vi "Agilent N6700 Series Read External Datalog.vi"() -> ()   [LabVIEW 2016]
doc: "Configures the external datalog then reads it from the instrument's buffer."
uses:
  <instrlib>/Agilent N6700 Series/Agilent N6700 Series.lvlib
panel:
  out "External Log":string
  in  "Max Records (10)":i32=10
  in  "Enable Minimum Maximum Log (False)":bool
  in  "Enable Data Log (True)":bool=TRUE
  in  "Data Log Period (0.1 s)":dbl=0.1
  in  "Data Log Auto Range (False)":bool=TRUE
  in  "Data Log Type (1: Voltage)":i32(ring)=1 items=["Voltage"=1, "Current"=0]
  in  "Channel Name (3)":string="3"
  in  "VISA resource name":refnum<visa-resource-name>
  # "(c) 2004-2019  National Instruments.  ALL RIGHTS RESERVED."
  # "Agilent N6700 DC Power Supply"
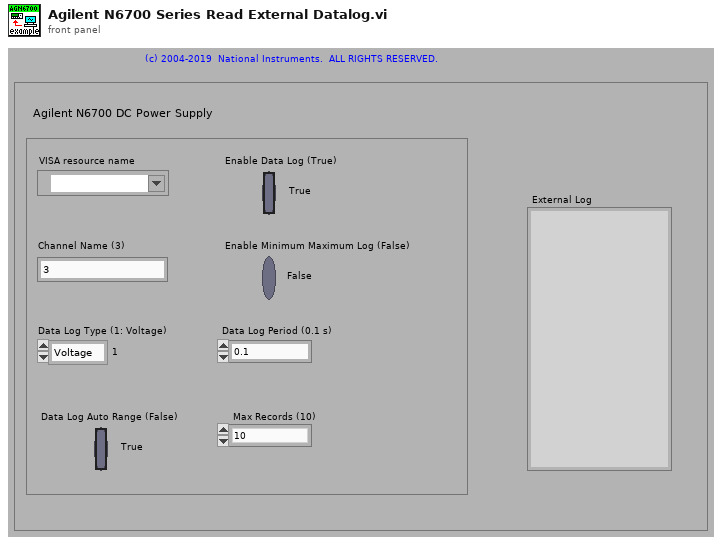
[diagram p1: front panel]
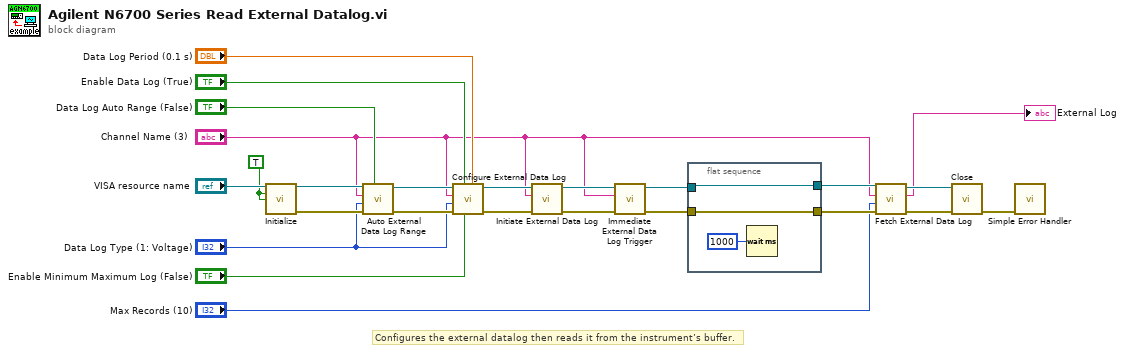
[diagram p0: block diagram]
diagram:
  w23 = TRUE ("Reset? (T: Yes)")
  # "Configures the external datalog then reads it from the instrument’s buffer."
  n1 = call <instrlib>:"Initialize.vi"("VISA resource name"="VISA resource name", "ID Query? (T: Yes)"=w23, "Reset? (T: Yes)"=w23) -> ("VISA resource name out"=w22:refnum<visa-resource-name>, "error out"=w21:errorcluster)  [unwired: 11 in]
  n2 = call <instrlib>:"Auto External Data Log Range.vi"("External Data Log Auto Range (False)"="Data Log Auto Range (False)", "error in (no error)"=w21, "External Data Log Type (1: Voltage)"="Data Log Type (1: Voltage)", "Channel Name (1)"="Channel Name (3)", "VISA resource name"=w22) -> ("error out"=w18:errorcluster, "VISA resource name out"=w19:refnum<visa-resource-name>)  [unwired: 5 in]
  n3 = call <instrlib>:"Configure External Data Log.vi"("External Data Log Period (0.1 s)"="Data Log Period (0.1 s)", "Enable Minimum Maximum Log (False)"="Enable Minimum Maximum Log (False)", "Enable External Data Log (False)"="Enable Data Log (True)", "error in (no error)"=w18, "External Data Log Type (1: Voltage)"="Data Log Type (1: Voltage)", "Channel Name (1)"="Channel Name (3)", "VISA resource name"=w19) -> ("error out"=w12:errorcluster, "VISA resource name out"=w13:refnum<visa-resource-name>)  [unwired: 3 in]
  n4 = call <instrlib>:"Initiate External Data Log.vi"("error in (no error)"=w12, "Channel Name (1)"="Channel Name (3)", "VISA resource name"=w13) -> ("error out"=w10:errorcluster, "VISA resource name out"=w11:refnum<visa-resource-name>)  [unwired: 7 in]
  n5 = call <instrlib>:"Immediate External Data Log Trigger.vi"("error in (no error)"=w10, "Channel Name (1)"="Channel Name (3)", "VISA resource name"=w11) -> ("error out"=w8:errorcluster, "VISA resource name out"=w9:refnum<visa-resource-name>)  [unwired: 7 in]
  n6 = flat-sequence {
    tunnel: w9 -> [w28]
    tunnel: [w28] -> w6
    tunnel: [w26] -> w7
    tunnel: w8 -> [w26]
    frame #0 {
      n7 = Wait (ms)(milliseconds to wait=u32 1000) -> ()  [unwired: 1 out]
    }
  }
  n8 = call <instrlib>:"Fetch External Data Log.vi"("error in (no error)"=w7, "Max Records (1)"="Max Records (10)", "Channel Name (1)"="Channel Name (3)", "VISA resource name"=w6) -> ("error out"=w2:errorcluster, "External Log"=→"External Log":string, "VISA resource name out"=w3:refnum<visa-resource-name>)  [unwired: 5 in]
  n9 = call <instrlib>:"Close.vi"("VISA resource name"=w3, "error in (no error)"=w2) -> ("error out"=w25:errorcluster)  [unwired: 13 in]
  n10 = call <vilib>:"Simple Error Handler.vi"("error in (no error)"=w25) -> ()  [unwired: 4 in, 5 out]
